vi "Build Attr Tree.vi"(7 "Flush Tree?":bool, 8 "error in (no error)":errorcluster, 9 "Filter":string="exposure trigger", 10 "Attr Infos":T1[](array[typedef]), 11 "Camera Settings Dialog in":refnum<class "Camera Settings Dialog.lvclass">) -> (0 "error out":errorcluster, 3 "Camera Settings Dialog out":refnum<class "Camera Settings Dialog.lvclass">)   [LabVIEW 2020, in "Camera Settings Dialog UI.lvlib" / "Camera Settings Dialog.lvclass"]
uses:
  Camera Settings Dialog.lvclass
  C:/Users/AlexK/work/LabVIEW Programme/HIJ_Vision_Project_LV2020/Submodules/Viewable Actor/ViewableActor/ViewableActor.lvclass
  Camera Attribute Info.ctl
  Viewable Actor/ViewableActor/ViewableActor.lvclass/ViewableActor.ctl
  Camera Settings Dialog.lvclass/Camera Settings Dialog.ctl
  Viewable Actor/ViewableActor/Read UI VI Ref.vi
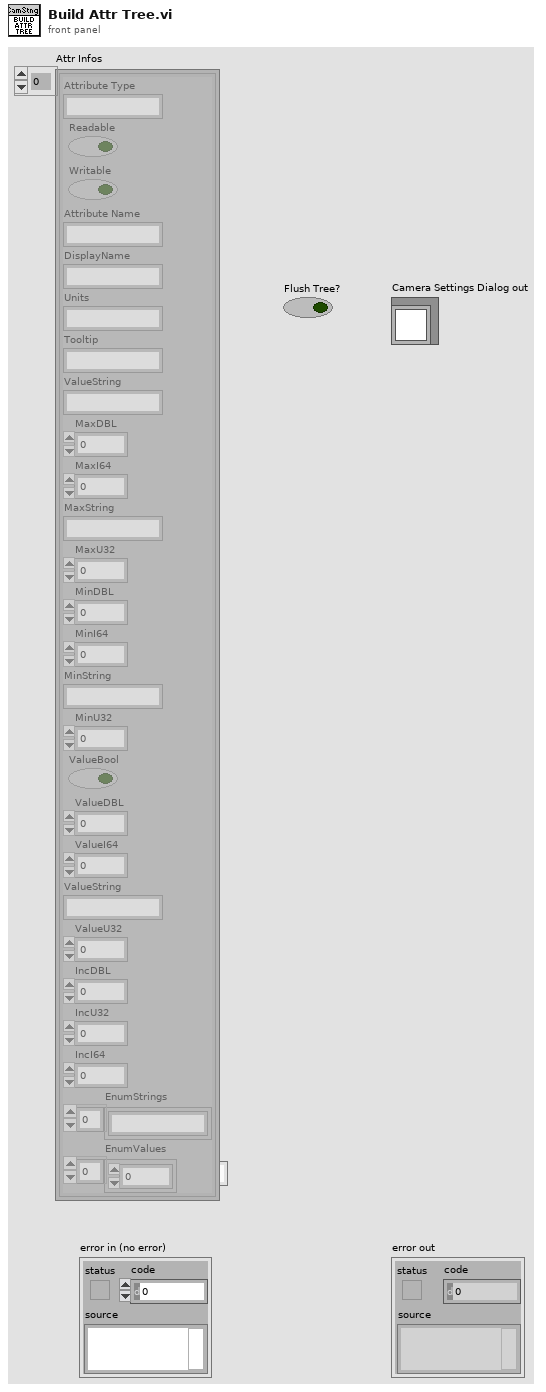
[diagram p1: front panel]
types:
  T1 = typedef "Camera Attribute Info.ctl" = cluster{"Attribute Type":string, "Readable":bool, "Writable":bool, "Attribute Name":string, "DisplayName":string, "Units":string, "Tooltip":string, "ValueString":string, "MaxDBL":dbl, "MaxI64":i64, "MaxString":string, "MaxU32":u32, "MinDBL":dbl, "MinI64":i64, "MinString":string, "MinU32":u32, "ValueBool":bool, "ValueDBL":dbl, "ValueI64 ":i64, "ValueString":string, "ValueU32":u32, "IncDBL":dbl, "IncU32":u32, "IncI64":i64, "EnumStrings":string[], "EnumValues":u32[]}
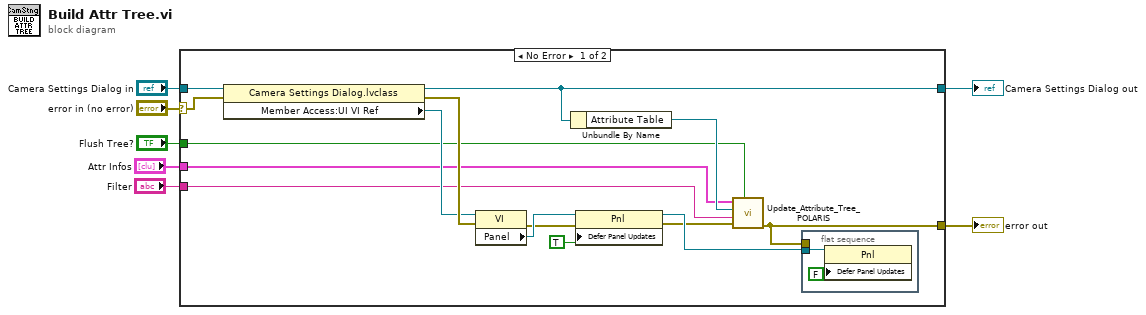
[diagram p0: block diagram]
diagram:
  n1 = case shown="No Error" "error in (no error)" {
    selector: "error in (no error)" -> [w12 w26]
    tunnel: [w8 w26] -> w6
    tunnel: [w15 w25] -> w4
    tunnel: "Camera Settings Dialog in" -> [w20 w25]
    tunnel: "Filter" -> [w13 _]
    tunnel: "Attr Infos" -> [w11 _]
    tunnel: "Flush Tree?" -> [w9 _]
    frame No Error {
      n2 = property class="Camera Settings Dialog.lvclass"(reference=w20, error in=w12) -> (reference out=w15:refnum<class "Camera Settings Dialog.lvclass">, error out=w22:errorcluster, "Member Access:UI VI Ref"=w16:refnum<vi>)
      n3 = property class="VI"(reference=w16, error in=w22) -> (error out=w10:errorcluster, "Panel"=w17:refnum<vi>)  [unwired: 1 out]
      n4 = Unbundle By Name(w15) -> ("Attribute Table"=w14:refnum<vi>)
      n5 = property class="Pnl"(reference=w17, error in=w10, "Defer Panel Updates"=TRUE) -> (reference out=w21:refnum<vi>, error out=w19:errorcluster)
      n6 = call "Update_Attribute_Tree_POLARIS.vi"("Flush Tree?"=w9, "error in"=w19, "Filter"=w13, "Tree Control In"=w14, "Attribute Information Array"=w11) -> ("error out"=w8:errorcluster)  [unwired: 3 in]
      n7 = flat-sequence {
        tunnel: w21 -> [w24]
        tunnel: w8 -> [_]
        frame #0 {
          n8 = property class="Pnl"(reference=w24, "Defer Panel Updates"=FALSE ("Flush Tree?")) -> ()  [unwired: 1 in, 2 out]
        }
      }
    }
    frame Error {
    }
  }
  "error out" <- w6
  "Camera Settings Dialog out" <- w4
